vi "Init.vi"(4 "Update delay (ms)":u32, 5 "Transparency":u8, 6 "Y offset":i32, 7 "X offset":i32, 8 "error in (no error)":errorcluster, 9 "WinHeight":u32, 10 "WinWidth":u32) -> (0 "error out":errorcluster, 3 "FolloWin out":refnum<class "FolloWin.lvclass">)   [LabVIEW 2023, in "FolloWin.lvclass"]
doc: "The Initialize method of the class FolloWin\n\n- instantiates an object. \n- writes all the control references of the FolloWin window into the object. \n- sets all its initial parameters.\n- setups the FolloWin window so it'll have that minimalist look - i.e. frame only"
uses:
  FolloWin.lvclass
  FolloWin.vi
  FolloWin.lvclass/FolloWin.ctl
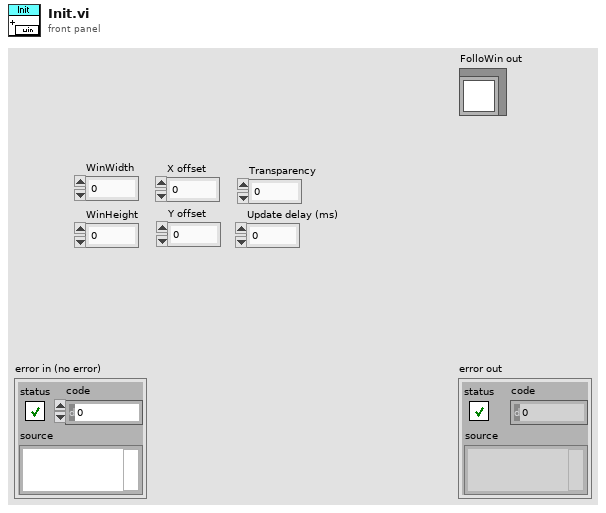
[diagram p1: front panel]
types:
  T1 = typedef "LVRectTypeDef.ctl" = cluster{"Left":i16, "Top":i16, "Right":i16, "Bottom":i16}
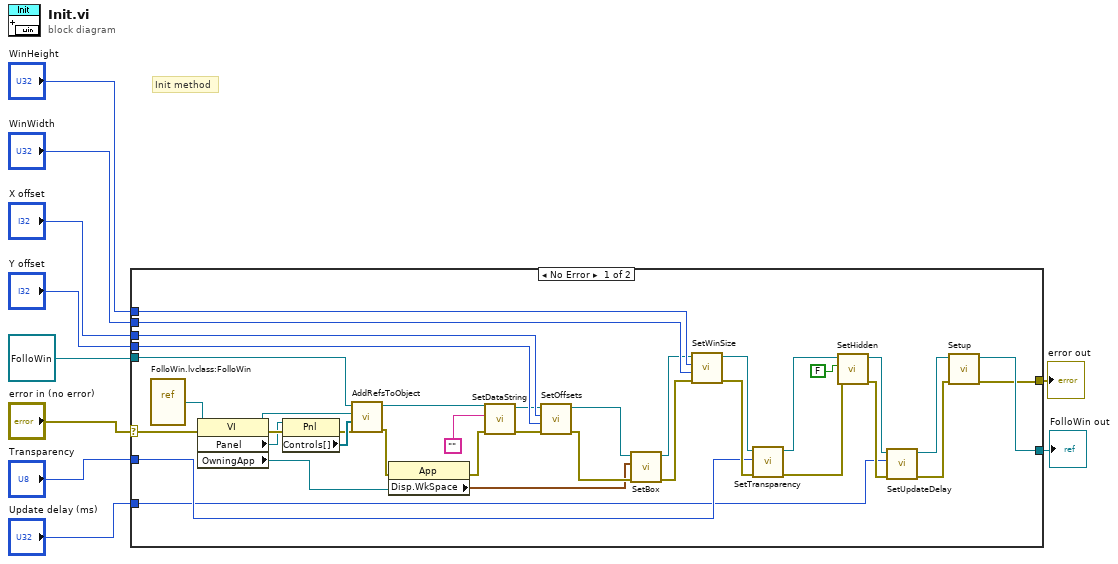
[diagram p0: block diagram]
diagram:
  # "Init method"
  n1 = case shown="No Error" "error in (no error)" {
    selector: "error in (no error)" -> [w44 w49]
    tunnel: [w24 w49] -> w9
    tunnel: [w26 w48] -> w7
    tunnel: refnum<class "FolloWin.lvclass"> refnum ("FolloWin in") -> [w22 w48]
    tunnel: "WinHeight" -> [w42 _]
    tunnel: "WinWidth" -> [w41 _]
    tunnel: "Y offset" -> [w38 _]
    tunnel: "X offset" -> [w37 _]
    tunnel: "Transparency" -> [w29 _]
    tunnel: "Update delay (ms)" -> [w28 _]
    frame No Error {
      n2 = vi-ref "FolloWin.lvclass:FolloWin.vi"() -> (w40:refnum<vi>)
      n3 = property on="Property Node" class="VI"(reference=w40, error in=w44) -> (reference out=w39:refnum<vi>, error out=w46:errorcluster, "Panel"=w43:refnum<vi>, "OwningApp"=w18:refnum<vi>)
      n4 = property on="Property Node" class="Pnl"(reference=w43, error in=w46) -> (error out=w45:errorcluster, "Controls[]"=w47:refnum<vi>[])  [unwired: 1 out]
      n5 = call "AddRefsToObject.vi"("error in (no error)"=w45, "Controls[]"=w47, "VI Refnum"=w39, "FolloWin in"=w22) -> ("error out"=w12:errorcluster, "FolloWin out"=w19:refnum<class "FolloWin.lvclass">)  [unwired: 6 in]
      n6 = property class="App"(reference=w18, error in=w12) -> (error out=w11:errorcluster, "Disp.WkSpace"=w13:T1)  [unwired: 1 out]
      n7 = call-dynamic "SetDataString.vi"("error in (no error)"=w11, "DataString"="", "FolloWin in"=w19) -> ("error out"=w21:errorcluster, "FolloWin out"=w20:refnum<class "FolloWin.lvclass">)  [unwired: 7 in]
      n8 = call-dynamic "SetOffsets.vi"("error in (no error)"=w21, "Y offset"=w38, "X offset"=w37, "FolloWin in"=w20) -> ("error out"=w17:errorcluster, "FolloWin out"=w15:refnum<class "FolloWin.lvclass">)  [unwired: 6 in]
      n9 = call "SetBox.vi"("error in (no error)"=w17, "Box"=w13, "FolloWin in"=w15) -> ("error out"=w16:errorcluster, "FolloWin out"=w14:refnum<class "FolloWin.lvclass">)  [unwired: 7 in]
      n10 = call-dynamic "SetWinSize.vi"("error in (no error)"=w16, "Width"=w41, "Height"=w42, "FolloWin in"=w14) -> ("error out"=w35:errorcluster, "FolloWin out"=w36:refnum<class "FolloWin.lvclass">)  [unwired: 6 in]
      n11 = call-dynamic "SetTransparency.vi"("error in (no error)"=w35, "Transparency"=w29, "FolloWin in"=w36) -> ("error out"=w33:errorcluster, "FolloWin out"=w34:refnum<class "FolloWin.lvclass">)  [unwired: 7 in]
      n12 = call-dynamic "SetHidden.vi"("error in (no error)"=w33, "Hidden?"=FALSE, "FolloWin in"=w34) -> ("error out"=w30:errorcluster, "FolloWin out"=w31:refnum<class "FolloWin.lvclass">)  [unwired: 7 in]
      n13 = call-dynamic "SetUpdateDelay.vi"("error in (no error)"=w30, "Update delay (ms)"=w28, "FolloWin in"=w31) -> ("error out"=w25:errorcluster, "FolloWin out"=w27:refnum<class "FolloWin.lvclass">)  [unwired: 7 in]
      n14 = call-dynamic "Setup.vi"("error in (no error)"=w25, "FolloWin in"=w27) -> ("error out"=w24:errorcluster, "FolloWin out"=w26:refnum<class "FolloWin.lvclass">)  [unwired: 8 in]
    }
    frame Error {
    }
  }
  "error out" <- w9
  "FolloWin out" <- w7
